vi "VBreak.vi"(2 "Condition d'arret":T1, 3 "Condition Initial":T2={"Range"=0.0, "Ilim"=0.0, "Level"=0.0, "Channel"=1, "Timed Totalize"=0.1} {"Channel" items=["Channel 1"=1, "Channel 2"=2]}) -> (0 "VBreak":dbl, 1 "Count":dbl)   [LabVIEW 2014]
uses:
  VBreakInitialCond.ctl
  VBreakStopCondition.ctl
  <instrlib>/Agilent 532XX Series/Public/Configure/Measurement/Configure Measurement (Totalize Timed).vi
  <instrlib>/Agilent 532XX Series/Public/Data/Read Measurement (Single).vi
  <instrlib>/Agilent 532XX Series/Agilent 532XX Series.lvlib
panel:
  in  "stop":bool
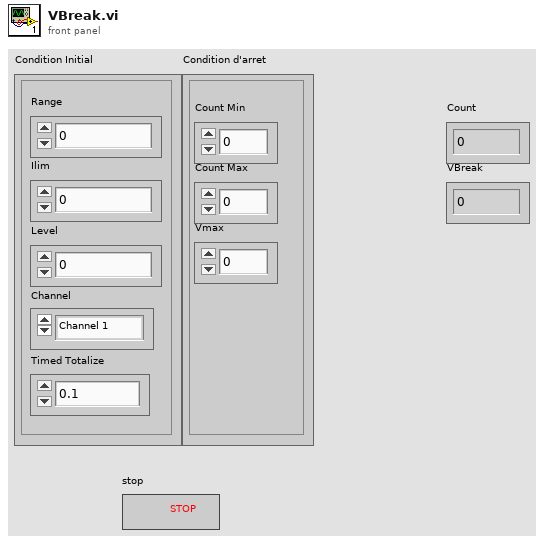
[diagram p1: front panel]
types:
  T1 = typedef "VBreakStopCondition.ctl" = cluster{"Count Min":dbl, "Count Max":dbl, "Vmax":dbl}
  T2 = typedef "VBreakInitialCond.ctl" = cluster{"Range":dbl, "Ilim":dbl, "Level":dbl, "Channel":i32, "Timed Totalize":dbl}
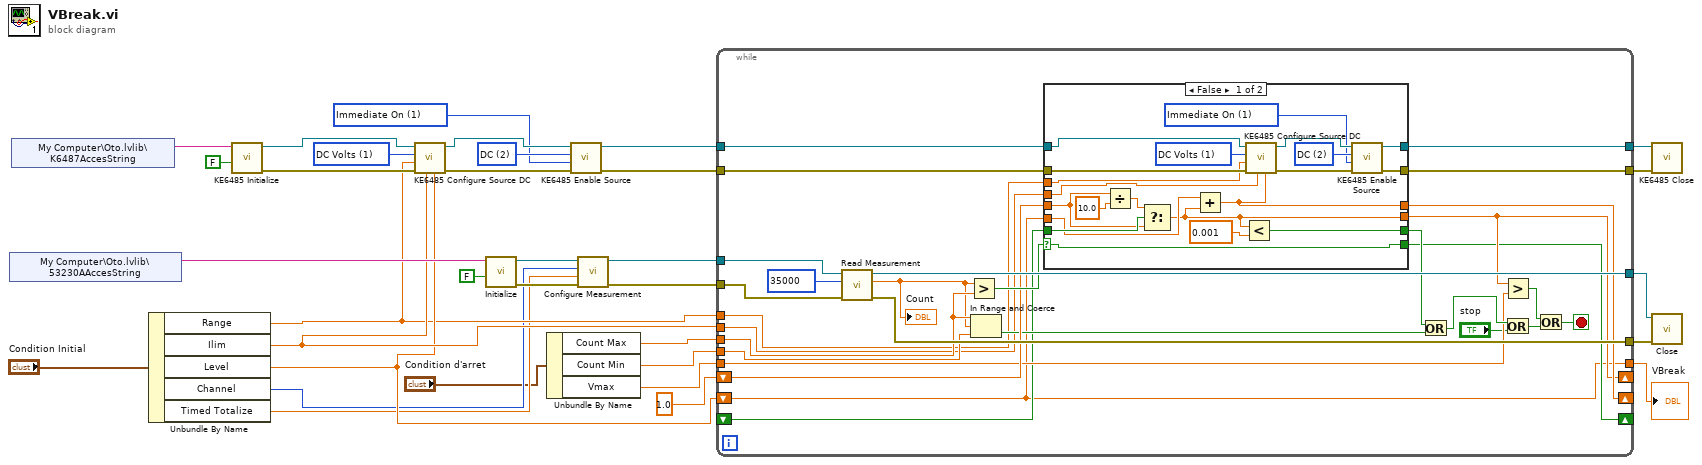
[diagram p0: block diagram]
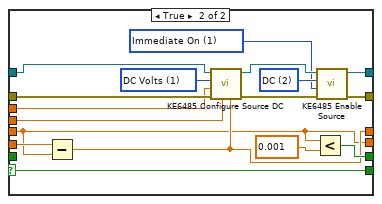
[diagram p2: hidden frame]
diagram:
  w19 = 1 items=["Immediate On"=1, "Immediate Off"=2, "Immediate Standby"=4, "Auto Sync Enabled"=65536, "Auto Sync Disabled"=131072] ("output action")
  w22 = 2 items=["Bias"=1, "DC"=2, "Ramp"=4] ("generator")
  w25 = 1 items=["DC Volts"=1] ("function")
  n1 = shared-variable "My Computer\\Oto.lvlib\\53230AAccesString"() -> (w12:string)  [unwired: 1 in, 1 out]
  n2 = shared-variable "My Computer\\Oto.lvlib\\K6487AccesString"() -> (w13:string)  [unwired: 1 in, 1 out]
  n3 = Unbundle By Name("Condition Initial") -> ("Range"=w8:dbl, "Ilim"=w10:dbl, "Level"=w9:dbl, "Channel"=w7:i32, "Timed Totalize"=w6:dbl)
  n4 = call <instrlib>:"KE6485 Initialize.vi"("reset device"=FALSE, "resource name"=w13) -> ("error out"=w26:errorcluster, "instrument handle out"=w27:refnum<k15>)  [unwired: 8 in]
  n5 = call <instrlib>:"KE6485 Configure Source DC.vi"("level"=w9, "compliance limit"=w10, "error in (no error)"=w26, "range"=w8, "function"=w25, "instrument handle"=w27) -> ("error out"=w23:errorcluster, "instrument handle out"=w24:refnum<k15>)  [unwired: 4 in]
  n6 = call <instrlib>:"Initialize.vi"("Reset (True)"=FALSE, "VISA resource name"=w12) -> ("error out"=w17:errorcluster, "VISA resource name out"=w18:refnum<visa-resource-name>)  [unwired: 8 in]
  n7 = Unbundle By Name("Condition d'arret") -> ("Count Max"=w4:dbl, "Count Min"=w3:dbl, "Vmax"=w2:dbl)
  n8 = call <instrlib>:"KE6485 Enable Source.vi"("error in (no error)"=w23, "output action"=w19, "generator"=w22, "instrument handle"=w24) -> ("error out"=w20:errorcluster, "instrument handle out"=w21:refnum<k15>)  [unwired: 6 in]
  n9 = call-poly <instrlib>:"Configure Measurement.vi"("error in (no error)"=w17, "Timed Totalize (0.1 s)"=w6, "Channel (1: Channel 1)"=w7, "VISA resource name"=w18) -> ("error out"=w15:errorcluster, "VISA resource name out"=w16:refnum<visa-resource-name>)  [unwired: 6 in]
  n10 = while {
    tunnel: w21 -> [w53]
    tunnel: [w49] -> w32
    tunnel: w20 -> [w52]
    tunnel: [w50] -> w31
    tunnel: [w61] -> w29
    tunnel: [w60] -> w28
    tunnel: w16 -> [w58]
    tunnel: w15 -> [w57]
    tunnel: w4 -> [w56]
    tunnel: w3 -> [w59]
    shift-right: [w45] -> _
    shift-left: 1.0 -> [w54]
    shift-right: [w51] -> _
    shift-left: w9 -> [w36]
    tunnel: w2 -> [w44]
    tunnel: w10 -> [w40]
    tunnel: w8 -> [w39]
    shift-right: [w38] -> _
    shift-left: _ -> [w37]
    tunnel: [w36] -> w1
    stop <- w41 stop-if-true
    n11 = call-poly <instrlib>:"Read Measurement.vi"("error in (no error)"=w57, "Timeout (10000 ms)"=u32 35000, "VISA resource name"=w58) -> ("error out"=w60:errorcluster, "Measurement"=w35:dbl, "VISA resource name out"=w61:refnum<visa-resource-name>)  [unwired: 6 in]
    "Count" <- w35
    n12 = Greater?(x=w35, y=w56) -> (0:w55:bool)
    n13 = In Range and Coerce(upper limit=w56, x=w35, lower limit=w59) -> (In Range?=w47:bool)  [unwired: 1 out]
    n14 = case shown="False" w55 {
      selector: w55 -> [w70 w94]
      tunnel: w54 -> [w67 w93]
      tunnel: w53 -> [w83 w97]
      tunnel: w52 -> [w82 w96]
      tunnel: w36 -> [w65 w100]
      tunnel: [w64 w93] -> w45
      tunnel: [w63 w95] -> w51
      tunnel: [w75 w84] -> w50
      tunnel: [w76 w85] -> w49
      tunnel: [w80 w98] -> w46
      tunnel: w40 -> [w72 w92]
      tunnel: w39 -> [w71 w91]
      tunnel: [w70 w94] -> w38
      tunnel: w37 -> [w69 _]
      frame False {
        w73 = 1 items=["Immediate On"=1, "Immediate Off"=2, "Immediate Standby"=4, "Auto Sync Enabled"=65536, "Auto Sync Disabled"=131072] ("output action")
        w74 = 2 items=["Bias"=1, "DC"=2, "Ramp"=4] ("generator")
        w79 = 1 items=["DC Volts"=1] ("function")
        n15 = Divide(x=w67, y=10.0) -> (x/y=w68:dbl)
        n16 = Select(t=w68, s=w69, f=w67) -> (s? t:f=w64:dbl)
        n17 = Add(x=w65, y=w64) -> (x+y=w63:dbl)
        n18 = Less?(x=w64, y=0.001) -> (x < y?=w80:bool)
        n19 = call <instrlib>:"KE6485 Configure Source DC.vi"("level"=w63, "compliance limit"=w72, "error in (no error)"=w82, "range"=w71, "function"=w79, "instrument handle"=w83) -> ("error out"=w77:errorcluster, "instrument handle out"=w78:refnum<k15>)  [unwired: 4 in]
        n20 = call <instrlib>:"KE6485 Enable Source.vi"("error in (no error)"=w77, "output action"=w73, "generator"=w74, "instrument handle"=w78) -> ("error out"=w75:errorcluster, "instrument handle out"=w76:refnum<k15>)  [unwired: 6 in]
      }
      frame True {
        w86 = 1 items=["Immediate On"=1, "Immediate Off"=2, "Immediate Standby"=4, "Auto Sync Enabled"=65536, "Auto Sync Disabled"=131072] ("output action")
        w87 = 2 items=["Bias"=1, "DC"=2, "Ramp"=4] ("generator")
        w90 = 1 items=["DC Volts"=1] ("function")
        n21 = Subtract(x=w100, y=w93) -> (x-y=w95:dbl)
        n22 = call <instrlib>:"KE6485 Configure Source DC.vi"("level"=w95, "compliance limit"=w92, "error in (no error)"=w96, "range"=w91, "function"=w90, "instrument handle"=w97) -> ("error out"=w88:errorcluster, "instrument handle out"=w89:refnum<k15>)  [unwired: 4 in]
        n23 = Less?(x=w93, y=0.001) -> (x < y?=w98:bool)
        n24 = call <instrlib>:"KE6485 Enable Source.vi"("error in (no error)"=w88, "output action"=w86, "generator"=w87, "instrument handle"=w89) -> ("error out"=w84:errorcluster, "instrument handle out"=w85:refnum<k15>)  [unwired: 6 in]
      }
    }
    n25 = Or(x=w46, y=w47) -> (x .or. y?=w48:bool)
    n26 = Greater?(x=w45, y=w44) -> (0:w43:bool)
    n27 = Or(x=w48, y="stop") -> (x .or. y?=w42:bool)
    n28 = Or(x=w43, y=w42) -> (x .or. y?=w41:bool)
  }
  "VBreak" <- w1
  n29 = call <instrlib>:"KE6485 Close.vi"("error in (no error)"=w31, "instrument handle"=w32) -> ()  [unwired: 9 in, 1 out]
  n30 = call <instrlib>:"Close.vi"("error in (no error)"=w28, "VISA resource name"=w29) -> ()  [unwired: 9 in, 1 out]
